vi "Set Color.vi"(8 "error in (no error)":errorcluster, 10 "Color":u32, 11 "object in":refnum<class "Game Component.lvclass">) -> (0 "error out":errorcluster, 3 "object out":refnum<class "Game Component.lvclass">)   [LabVIEW 2017, in "Game Component.lvclass"]
uses:
  Game Component.lvclass
  Game Component.lvclass/Game Component.ctl
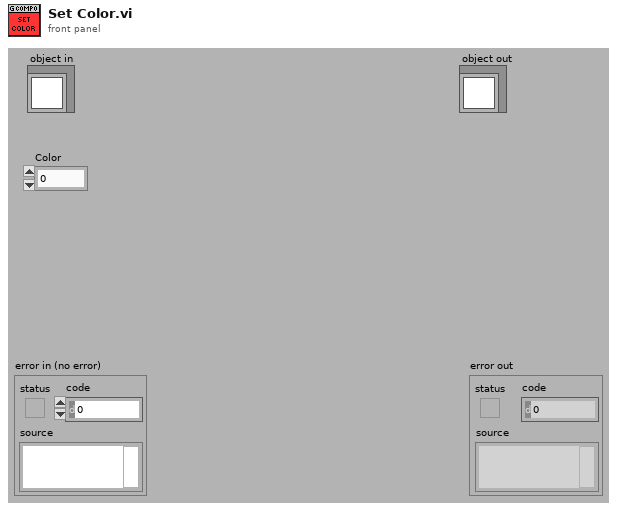
[diagram p1: front panel]
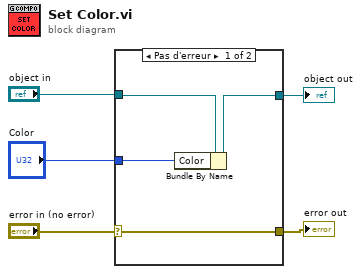
[diagram p0: block diagram]
diagram:
  n1 = case shown="Pas d'erreur" "error in (no error)" {
    selector: "error in (no error)" -> [w8 w11]
    tunnel: [w8 w11] -> w4
    tunnel: [w6 w10] -> w2
    tunnel: "object in" -> [w7 w10]
    tunnel: "Color" -> [w9 _]
    frame No Error {
      n2 = Bundle By Name(cluster=w7, "Color"=w9) -> (w6:refnum<class "Game Component.lvclass">)
    }
    frame Error {
    }
  }
  "error out" <- w4
  "object out" <- w2
